vi "ApplyLibIconOverlayToVIIcon.vi"(4 "External User Layer":refnum<class "Layer.lvclass">[](array[class]), 6 "Add ext user layer? (F)":bool, 7 "Lib Refnum":refnum<vi>, 8 "Don't consider curr VI Icon? (F)":bool, 9 "overlay image":T8={"image type"=0, "image depth"=0, "image"=[], "mask"=[], "colors"=[], "Rectangle"={"left"=0, "top"=0, "right"=32, "bottom"=32}}, 10 "overlay provided?":bool, 11 "VI Refnum":refnum<vi>) -> (0 "Error code out":i32)   [LabVIEW 2021]
uses:
  <vilib>/picture/picture.llb/imagedata.ctl
  Controls/IE Data.ctl
  Class/Ants/Ants.lvclass
  Class/FakedArray/FakedArray.lvclass
  vi.lib/LabVIEW Icon API/lv_icon/Classes/Icon/Icon.lvclass
  Class/Icon Library/Glyph.lvclass
  Class/Settings/Settings.lvclass
  Class/Tools/Tools Paint.lvclass
  Controls/IE Classes.ctl
  Controls/References Cluster.ctl
  Controls/SupportClass.ctl
  <vilib>/Utility/miscctls.llb/LVPoint32TypeDef.ctl
  Controls/SupportClass_Action.ctl
  vi.lib/LabVIEW Icon API/lv_icon/Controls/IEColor.ctl
  vi.lib/LabVIEW Icon API/lv_icon/Classes/Layer/Layer.lvclass
  vi.lib/LabVIEW Icon API/lv_icon/Controls/Layer.ctl
  vi.lib/LabVIEW Icon API/lv_icon/Controls/Graphic.ctl
  vi.lib/LabVIEW Icon API/lv_icon/lv_icon.lvlib
  vi.lib/LabVIEW Icon API/lv_icon/Classes/Icon Framework/Icon Framework.lvclass
panel:
  in  "Data in":T1={"Class"={"Ants"=refnum, "Layer"=refnum, "Templates"=refnum, "Icon"=refnum, "Glyph"=refnum, "Settings"=refnum, "Tools"=refnum}, "Ref"={"Add Layer"=refnum, "Remove Layer"=refnum, "Line Text"=[], "Body Text Spec"=refnum, "DNL_Font"=refnum, "glyph path str"=refnum, "templates path str"=refnum, "Arrow Up"=refnum, "Arrow Down"=refnum, "IE VI Ref"=refnum, "Glyphs tree"=refnum, "Templates tree"=refnum, "Layer Icon Text"=refnum, "Layer Template"=refnum, "Clipboard"=refnum, "BW icon in"=refnum, "Color icon in"=refnum, "Layer Clust"=refnum, "Body Text"=refnum, "DNL_Framework Templates"=refnum, "Search Templates"=refnum, "TextMarker"=refnum, "Tab Control"=refnum, "Search Glyphs"=refnum, "Line Color"=refnum, "DNL_Glyphs []"=refnum, "Fill Color"=refnum, "Tools"=refnum, "Glyphs tree"=refnum, "Icon"=refnum, "Preview"=refnum, "Ants"=refnum, "Terminals"=refnum, "menu reference"=refnum, "LayerNames"=[], "GlyphLoadAnimation"=refnum, "TemplateLoadAnimation"=refnum, "refreshGlyphs"=refnum, "refreshTemplates"=refnum}, "Support"={"AntsRect"={"left"=0, "top"=0, "right"=0, "bottom"=0}, "Mouse Move Coords"={"Horizontal"=0, "Vertical"=0}, "Mouse Down Coords"={"Horizontal"=0, "Vertical"=0}, "Temp Coord"={"Horizontal"=0, "Vertical"=0}, "Action"=enum."Default", "Edge Color"=4914962, "Fill Color"=16860, "Mouse Down?"=FALSE, "Draft Mode?"=FALSE, "Temp Icon"=bytes[3102], "CTRL Pressed"=FALSE, "Move Selection?"=FALSE, "AntsRect Orig"={"left"=0, "top"=0, "right"=0, "bottom"=0}, "Text"="", "TM Set?"=FALSE, "Mouse inside icon?"=FALSE, "Tool (old value)"=0, "Pencil Move Color"=0, "Swap Colors?"=FALSE, "Shift pressed?"=FALSE}}
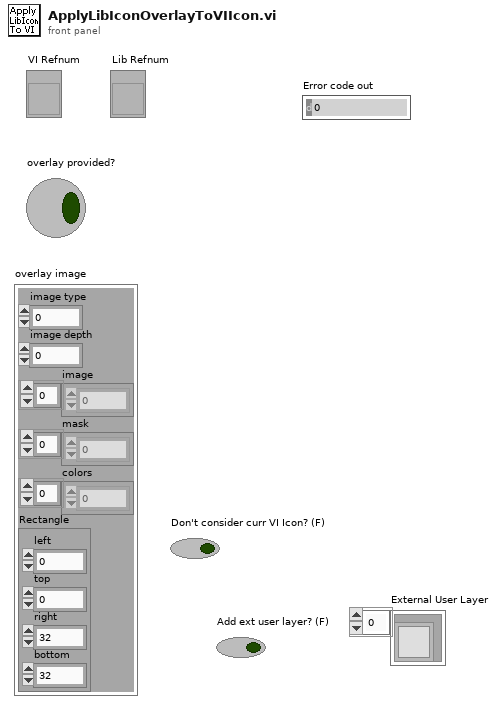
[diagram p1: front panel]
types:
  T1 = typedef "IE Data.ctl" = cluster{"Class":T2, "Ref":T3, "Support":T4}
  T2 = typedef "IE Classes.ctl" = cluster{"Ants":refnum<class "Ants.lvclass">, "Layer":refnum<class "FakedArray.lvclass">, "Templates":refnum<class "FakedArray.lvclass">, "Icon":refnum<class "Icon.lvclass">, "Glyph":refnum<class "Glyph.lvclass">, "Settings":refnum<class "Settings.lvclass">, "Tools":refnum<class "Tools Paint.lvclass">}
  T3 = typedef "References Cluster.ctl" = cluster{"Add Layer":refnum<vi>, "Remove Layer":refnum<vi>, "Line Text":refnum<vi>[], "Body Text Spec":refnum<vi>, "DNL_Font":refnum<vi>, "glyph path str":refnum<vi>, "templates path str":refnum<vi>, "Arrow Up":refnum<vi>, "Arrow Down":refnum<vi>, "IE VI Ref":refnum<vi>, "Glyphs tree":refnum<vi>, "Templates tree":refnum<vi>, "Layer Icon Text":refnum<vi>, "Layer Template":refnum<vi>, "Clipboard":refnum<vi>, "BW icon in":refnum<vi>, "Color icon in":refnum<vi>, "Layer Clust":refnum<vi>, "Body Text":refnum<vi>, "DNL_Framework Templates":refnum<vi>, "Search Templates":refnum<vi>, "TextMarker":refnum<vi>, "Tab Control":refnum<vi>, "Search Glyphs":refnum<vi>, "Line Color":refnum<vi>, "DNL_Glyphs []":refnum<vi>, "Fill Color":refnum<vi>, "Tools":refnum<vi>, "Glyphs tree":refnum<vi>, "Icon":refnum<vi>, "Preview":refnum<vi>, "Ants":refnum<vi>, "Terminals":refnum<vi>, "menu reference":refnum<k9>, "LayerNames":refnum<vi>[], "GlyphLoadAnimation":refnum<vi>, "TemplateLoadAnimation":refnum<vi>, "refreshGlyphs":refnum<vi>, "refreshTemplates":refnum<vi>}
  T4 = typedef "SupportClass.ctl" = cluster{"AntsRect":cluster{"left":i16, "top":i16, "right":i16, "bottom":i16}, "Mouse Move Coords":T5, "Mouse Down Coords":T5, "Temp Coord":T5, "Action":T6, "Edge Color":T7, "Fill Color":T7, "Mouse Down?":bool, "Draft Mode?":bool, "Temp Icon":picture, "CTRL Pressed":bool, "Move Selection?":bool, "AntsRect Orig":cluster{"left":i16, "top":i16, "right":i16, "bottom":i16}, "Text":string, "TM Set?":bool, "Mouse inside icon?":bool, "Tool (old value)":u32, "Pencil Move Color":u32, "Swap Colors?":bool, "Shift pressed?":bool}
  T5 = typedef "LVPoint32TypeDef.ctl" = cluster{"Horizontal":i32, "Vertical":i32}
  T6 = typedef "SupportClass_Action.ctl" = enum16{"Default", "Move Selection", "Glyph Library", "Tool"}
  T7 = typedef "IEColor.ctl" = u32
  T8 = typedef "imagedata.ctl" = cluster{"image type":i32, "image depth":i32, "image":u8[], "mask":u8[], "colors":u32[], "Rectangle":cluster{"left":i16, "top":i16, "right":i16, "bottom":i16}}
  T9 = typedef "Graphic.ctl" = cluster{"Rectangle":cluster{"left":i16, "top":i16, "right":i16, "bottom":i16}, "Path":path, "Image":picture, "Filter":string, "FileName":string}
  T10 = typedef "Layer.ctl" = cluster{"LayerIcon":picture, "LayerName":string, "Opacity":u8, "Visibility?":bool}
  T11 = typedef "INI.ctl" = cluster{"Show Layer Tab?":bool, "Show Terminals?":bool, "Text":cluster{"Font":T12, "Alignment":T13, "Size":T14}, "3rd party Templates":cluster{"Store 3rd party Templates?":bool, "Folder Name":string}, "Merge user layers on commit":bool, "Body Text":T15, "Fill Color":T7, "Edge Color":T7, "Tab":u16, "Tool":T16, "Disable Layers?":bool}
  T12 = typedef "Font.ctl" = string
  T13 = typedef "Alignment.ctl" = u16
  T14 = typedef "Font Size.ctl" = u8
  T15 = typedef "BodyText.ctl" = cluster{"Line 1 text":string, "Line 2 text":string, "Line 3 text":string, "Line 4 text":string, "Line 1 color":u32, "Line 2 color":u32, "Line 3 color":u32, "Line 4 color":u32, "Body Text Spec":cluster{"Font":T12, "Alignment":T13, "Size":u8}, "Center text vertically":bool, "Capitalize Text":bool}
  T16 = typedef "Tools.ctl" = enum32{"Pencil", "Line", "Dropper", "Fill", "Rectangle", "Filled Rectangle", "Ellipse", "Filled Ellipse", "Eraser", "Text", "Select", "Move"}
  T17 = typedef "LabVIEW Icon Stored Information.ctl" = cluster{"Text Visible?":bool, "Text Opacity":u8, "Templ Visible?":bool, "Templ Opacity":u8, "Relative Path from 1 to 2":path, "Image":picture, "All User Layers":refnum<class "Layer.lvclass">[], "Body Text":T15}
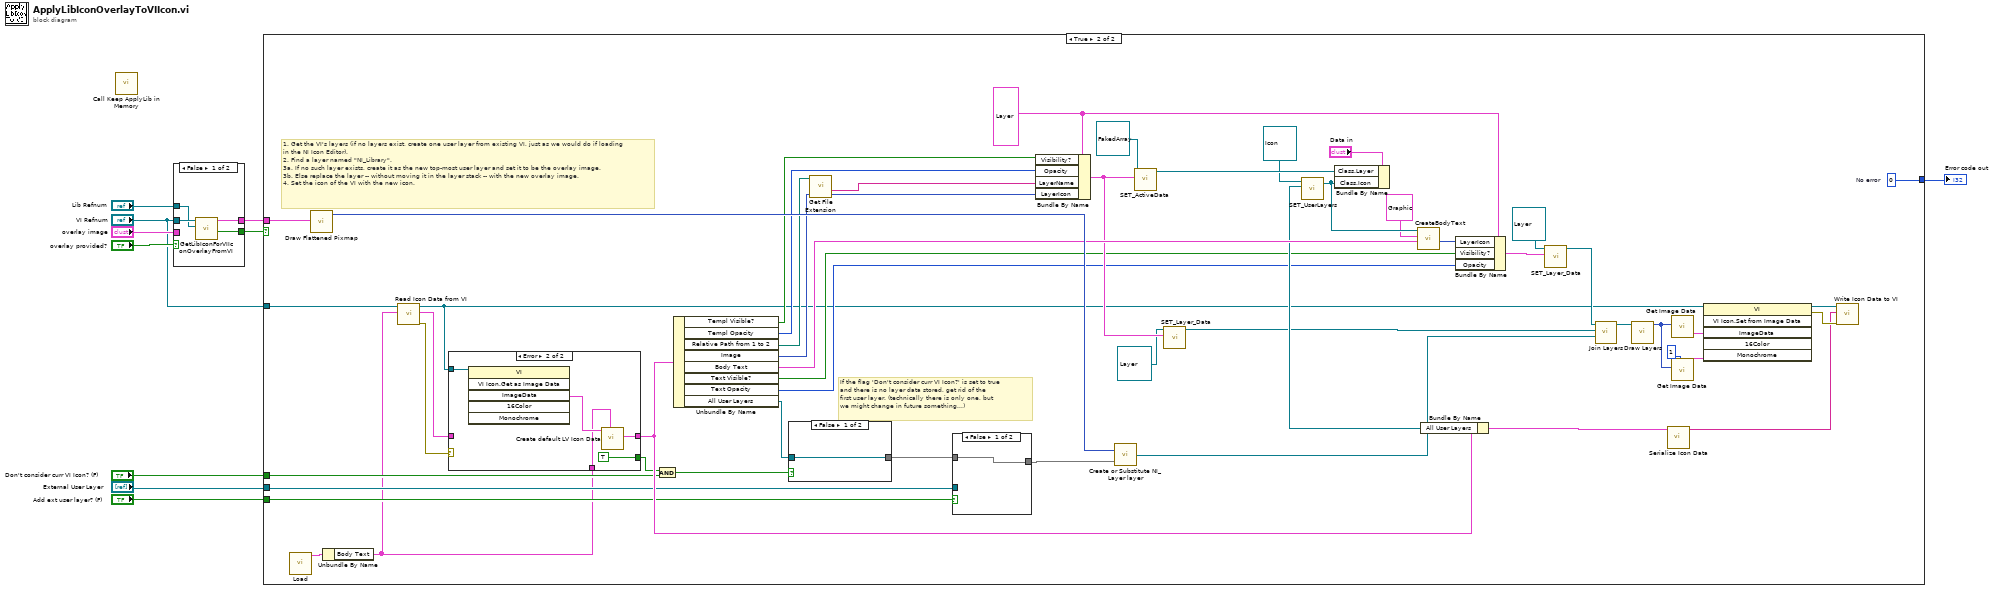
[diagram p0: block diagram]
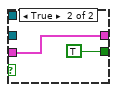
[diagram p2: hidden frame]
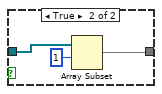
[diagram p4: hidden frame]
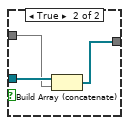
[diagram p5: hidden frame]
diagram:
  n1 = call "Call Keep ApplyLib in Memory.vi"() -> ()  [unwired: 1 out]
  n2 = case shown="False" "overlay provided?" {
    tunnel: "VI Refnum" -> [w14 _]
    tunnel: [w13 TRUE ("Owned by library?")] -> w10
    tunnel: [w12 w16] -> w9
    tunnel: "overlay image" -> [_ w16]
    tunnel: "Lib Refnum" -> [w11 _]
    frame False {
      n3 = call "GetLibIconForVIIconOverlayFromVI.vi"("Lib Refnum"=w11, "VI Refnum"=w14) -> ("Owned by library?"=w13:bool, "Library Icon For VI Overlay"=w12:T8)  [unwired: 8 out]
    }
    frame True {
    }
  }
  n4 = case shown="True" w10 {
    tunnel: w9 -> [_ w65]
    tunnel: [_ w66] -> w6
    tunnel: "VI Refnum" -> [_ w21]
    tunnel: "Add ext user layer? (F)" -> [_ w35]
    tunnel: "External User Layer" -> [_ w34]
    tunnel: "Don't consider curr VI Icon? (F)" -> [_ w33]
    frame False {
      # "No work needs to be done. VI is not owned by a library."
    }
    frame True {
      w40 = T10 {"LayerIcon"=bytes[3102], "LayerName"="", "Opacity"=100, "Visibility?"=TRUE} ("Data")
      w66 = 0  # No error
      # "If the flag 'Don't consider curr VI Icon?' is set to true\nand there is no layer data stored, get rid of the\nfirst user layer. (technically there is only one, but\nwe might change in future something...)"
      # "1. Get the VI's layers (if no layers exist, create one user layer from existing VI, just as we would do if loading in the NI Icon Editor).\n2. Find a layer named \"NI_Library\".\n3a. If no such layer exists, create it as the new top-most user layer and set it to be the overlay image.\n3b. Else replace the layer -- without moving it in the layer stack -- with the new overlay image.\n4. Set the icon of the VI with the new icon."
      n5 = call "Load.vi"() -> ("INI Data"=w28:T11)  [unwired: 2 in, 9 out]
      n6 = call <vilib>:"Draw Flattened Pixmap.vi"("image data"=w65) -> ("new picture"=w64:picture)  [unwired: 1 in, 7 out]
      n7 = Unbundle By Name(w28) -> ("Body Text"=w18:T15)
      n8 = call "Read Icon Data from VI.vi"("Default body text"=w18, "VI Ref in"=w21) -> ("error out"=w17:errorcluster, "Data"=w19:T17, "VI Ref out"=w20:refnum<vi>)  [unwired: 7 in]
      n9 = case shown="Error" w17 {
        tunnel: w19 -> [w75 _]
        tunnel: [w75 w77] -> w60
        tunnel: w20 -> [_ w80]
        tunnel: [_ TRUE] -> w32
        tunnel: w18 -> [_ w76]
        frame No Error {
        }
        frame Error {
          n10 = invoke class="VI" method="VI Icon.Get as Image Data"(reference=w80) -> ("ImageData"=w78:T8)  [unwired: 5 in, 5 out]
          n11 = call "Create default LV Icon Data.vi"("Body Text"=w76, "Pic Data in"=w78) -> ("VI Icon Data out"=w77:T17)  [unwired: 8 in, 1 out]
        }
      }
      n12 = And(x=w32, y=w33) -> (x .and. y?=w30:bool)
      n13 = Unbundle By Name(w60) -> ("Templ Visible?"=w57:bool, "Templ Opacity"=w56:u8, "Relative Path from 1 to 2"=w55:path, "Image"=w52:picture, "Body Text"=w53:T15, "Text Visible?"=w39:bool, "Text Opacity"=w38:u8, "All User Layers"=w31:refnum<class "Layer.lvclass">[])
      n14 = case shown="False" w30 {
        tunnel: w31 -> [w67 w70]
        tunnel: [w67 w68] -> w29
        frame False {
        }
        frame True {
          n15 = Array Subset(array=w70, index=1) -> (w68:refnum<class "Layer.lvclass">[])  [unwired: 1 in]
        }
      }
      n16 = call <vilib>:"Get File Extension.vi"("file"=w55) -> ("filename without extension"=w54:string)  [unwired: 6 in, 4 out]
      n17 = case shown="False" w35 {
        tunnel: w29 -> [w71 w73]
        tunnel: [w71 w72] -> w36
        tunnel: w34 -> [_ w74]
        frame False {
        }
        frame True {
          n18 = Build Array (concatenate)(w74, w73) -> (w72:refnum<class "Layer.lvclass">[])
        }
      }
      n19 = Bundle By Name(cluster=w40, "Visibility?"=w57, "Opacity"=w56, "LayerName"=w54, "LayerIcon"=w52) -> (w48:T10)
      n20 = call "Create or Substitute NI_Layer layer.vi"("All Layers in"=w36, "new picture"=w64) -> ("All Layers out"=w49:refnum<class "Layer.lvclass">[])
      n21 = call-dynamic "SET_ActiveData.vi"("Active Data"=w48, "FakedArray.lvclass in"=refnum<class "FakedArray.lvclass"> refnum) -> ("FakedArray.lvclass out"=w58:refnum<class "FakedArray.lvclass">)  [unwired: 8 in, 1 out]
      n22 = call-dynamic "SET_Layer_Data.vi"("Data"=w48, "Layer.lvclass in"=refnum<class "Layer.lvclass"> refnum) -> ("Layer.lvclass out"=w46:refnum<class "Layer.lvclass">)  [unwired: 8 in, 1 out]
      n23 = call-dynamic "SET_UserLayers.vi"("Layers"=w49, "Icon.lvclass in"=refnum<class "Icon.lvclass"> refnum) -> ("Icon.lvclass out"=w27:refnum<class "Icon.lvclass">)  [unwired: 8 in, 1 out]
      n24 = Bundle By Name(cluster="Data in", "Class.Layer"=w58, "Class.Icon"=w27) -> ()  [unwired: 1 out]
      n25 = call "CreateBodyText.vi"("Body Text"=w53, "Path and Icon Template"=T9 {"Rectangle"={"left"=0, "top"=0, "right"=0, "bottom"=0}, "Path"=path "", "Image"=bytes[0], "Filter"="", "FileName"=""}, "Icon.lvclass in"=w27) -> ("Body Text"=w42:picture)  [unwired: 1 in, 7 out]
      n26 = Bundle By Name(cluster=w60, "All User Layers"=w49) -> (w25:T17)
      n27 = Bundle By Name(cluster=w40, "LayerIcon"=w42, "Visibility?"=w39, "Opacity"=w38) -> (w41:T10)
      n28 = call-dynamic "SET_Layer_Data.vi"("Data"=w41, "Layer.lvclass in"=refnum<class "Layer.lvclass"> refnum) -> ("Layer.lvclass out"=w37:refnum<class "Layer.lvclass">)  [unwired: 8 in, 1 out]
      n29 = call "Join Layers.vi"("User Layers"=w49, "Template"=w46, "Icon Text"=w37) -> ("Layer out"=w45:refnum<class "Layer.lvclass">[])  [unwired: 3 in, 5 out]
      n30 = call "Draw Layers.vi"("Layers"=w45) -> ("Picture"=w44:picture)  [unwired: 4 in, 6 out]
      n31 = call "Serialize Icon Data.vi"("Icon data"=w25) -> ("data string"=w23:string)  [unwired: 9 in, 1 out]
      n32 = call "Get Image Data.vi"("Pic In"=w44) -> ("image data out"=w62:T8)  [unwired: 2 in, 8 out]
      n33 = call "Get Image Data.vi"("depth (24)"=1 ("depth"), "Pic In"=w44) -> ("image data out"=w61:T8)  [unwired: 2 in, 7 out]
      n34 = invoke class="VI" method="VI Icon.Set from Image Data"(reference=w20, "ImageData"=w62, "Monochrome"=w61) -> (reference out=w22:refnum<vi>, error out=w24:errorcluster)  [unwired: 3 in, 4 out]
      n35 = call "Write Icon Data to VI.vi"("error in (no error)"=w24, "Data"=w23, "VI Ref in"=w22) -> ()  [unwired: 7 in, 2 out]
    }
  }
  "Error code out" <- w6
